vi "Rec Targeting.vi"() -> ()   [LabVIEW 2012]
panel:
  in  "Y Motor":dbl
  in  "X Motor":dbl
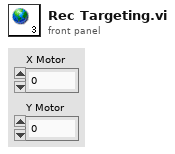
[diagram p1: front panel]
diagram:
